vi "myRIO_BRig_RT__Case_Exp_State_initTrial_dispense_pre.vi"(0 "input_dataMTrig":u16[](array[numeric]), 2 "Solenoid_Tcycle_L":u16=300, 3 "Solenoid_Tcycle_R":u16=300) -> (20 "output_dataMTrig":u16[](array[numeric]), 21 "output_state":T1)   [LabVIEW 2014]
uses:
  myRIO_Gil_RT_v1__states.vi
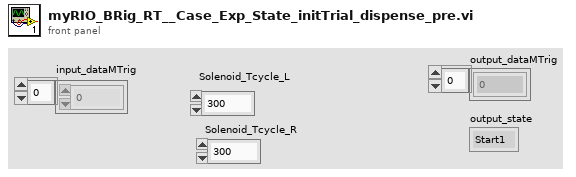
[diagram p1: front panel]
types:
  T1 = typedef "myRIO_Gil_RT_v1__states.vi" = enum16{"Start1", "Start2", "Start3", "initBlock", "initTrial", "initTrial_dispense_pre", "initTrial_dispense", "ENL1_pre", "ENL1", "ENL1Penalty_pre", "ENL1Penalty", "ENL2_pre", "ENL2", "ENL2Penalty_pre", "ENL2Penalty", "Cue1_pre", "Cue1", "Cue1Penalty_pre", "Cue1Penalty", "Cue2_pre", "Cue2", "Cue2Penalty_pre", "Cue2Penalty", "Selection_pre", "Selection", "SelectReward_pre", "SelectReward", "SelectRewardPost_pre", "SelectRewardPost", "SelectWrong_pre", "SelectWrong", "SelectTimeout_pre", "SelectTimeout", "SelectTimeout_post", "endTrial1", "endTrial2", "transferCheck", "transferPrepare", "transferCleanUp", "endBlock", "endExp"}
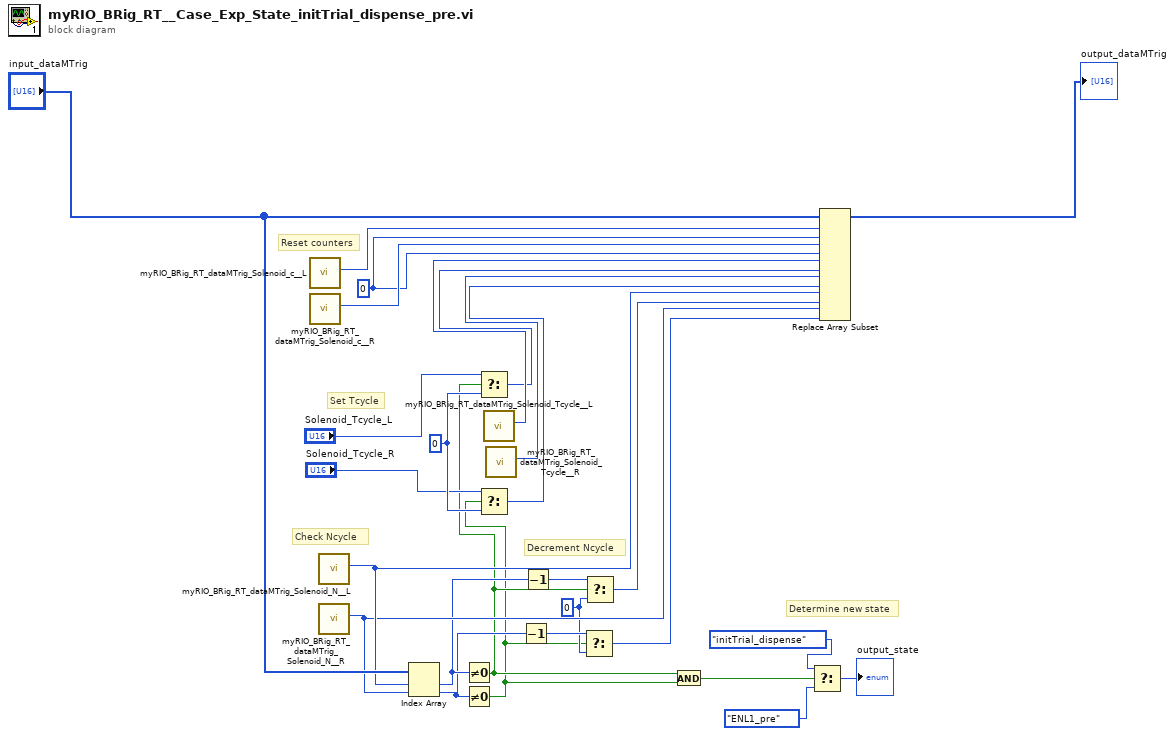
[diagram p0: block diagram]
diagram:
  w8 = u16 0 ("f")
  w22 = u16 0 ("f")
  w23 = u16 0 ("new element/subarray")
  # "Determine new state"
  # "Decrement Ncycle"
  # "Check Ncycle"
  # "Set Tcycle"
  # "Reset counters"
  n1 = call "myRIO_BRig_RT_dataMTrig_Solenoid_c__L.vi"() -> ("output_Solenoid_c__L"=w25:i32)  [unwired: 11 in]
  n2 = call "myRIO_BRig_RT_dataMTrig_Solenoid_c__R.vi"() -> ("output_Solenoid_c__R"=w24:i32)  [unwired: 11 in]
  n3 = call "myRIO_BRig_RT_dataMTrig_Solenoid_N__L.vi"() -> ("output_Solenoid_N__L"=w14:i32)  [unwired: 11 in]
  n4 = call "myRIO_BRig_RT_dataMTrig_Solenoid_N__R.vi"() -> ("output_Solenoid_N__R"=w13:i32)  [unwired: 11 in]
  n5 = Index Array(array="input_dataMTrig", index #1=w14, index #2=w13) -> (element #1=w12:u16, element #2=w10:u16)
  n6 = Not Equal To 0?(x=w12) -> (x != 0?=w5:bool)
  n7 = Not Equal To 0?(x=w10) -> (x != 0?=w4:bool)
  n8 = Select(t="Solenoid_Tcycle_L", s=w5, f=w22) -> (s? t:f=w18:u16)
  n9 = Select(t="Solenoid_Tcycle_R", s=w4, f=w22) -> (s? t:f=w16:u16)
  n10 = call "myRIO_BRig_RT_dataMTrig_Solenoid_Tcycle__L.vi"() -> ("output_Solenoid_Tcycle__L"=w19:i32)  [unwired: 11 in]
  n11 = call "myRIO_BRig_RT_dataMTrig_Solenoid_Tcycle__R.vi"() -> ("output_Solenoid_Tcycle__R"=w17:i32)  [unwired: 11 in]
  n12 = Decrement(x=w10) -> (x-1=w9:u16)
  n13 = Decrement(x=w12) -> (x-1=w11:u16)
  n14 = Select(t=w9, s=w4, f=w8) -> (s? t:f=w6:u16)
  n15 = Select(t=w11, s=w5, f=w8) -> (s? t:f=w7:u16)
  n16 = And(x=w5, y=w4) -> (x .and. y?=w15:bool)
  n17 = Select(t=myRIO_Gil_RT_v1__states.vi."initTrial_dispense", s=w15, f=myRIO_Gil_RT_v1__states.vi."ENL1_pre") -> (s? t:f=→"output_state":T1)
  n18 = Replace Array Subset(array="input_dataMTrig", new element #1=w23, index #1=w25, new element #2=w23, index #2=w24, new element #3=w18, index #3=w19, new element #4=w16, index #4=w17, new element #5=w7, index #5=w14, new element #6=w6, index #6=w13) -> (→"output_dataMTrig":u16[])
